vi "Select Channels and Update Properties.vi"(7 "guids":string[](array[string])=["4b95dee7-8d64-48ce-932c-f5fdd14e4d4c", "94e87467-031b-484c-a85e-bcbac581524d"], 8 "error in (no error)":errorcluster, 11 "Node Ptr":u64) -> (0 "error out":errorcluster)   [LabVIEW 2019, in "Protection and Counter Support System Explorer.lvlib"]
uses:
  Protection and Counter Support System Explorer.lvlib
  <vilib>/NI VeriStand/Custom Device Tools/Custom Device Utility Library/Custom Device Utility Library.lvlib
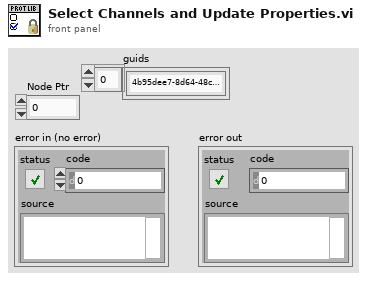
[diagram p1: front panel]
types:
  T1 = typedef "Protection and Counter Support System Explorer.lvlib/Protection Signal Settings.ctl" = cluster{"Input Channels":T2[], "Protection Type":T4}
  T2 = typedef "Protection and Counter Support System Explorer.lvlib/Protection Signal Linked Channel.ctl" = cluster{"Node Ref":T3}
  T3 = typedef "Custom Device API.lvlib/Custom Device Item Ref.ctl" = u64
  T4 = typedef "Protection and Counter Support Shared.lvlib/Protection Type.ctl" = enum16{"Arb ID + Bytes Checksum with Inversion", "Arb ID + Bytes CRC with Inversion", "Reversed Raw Signal Checksum with Inversion", "Concatenated Two's Compliment"}
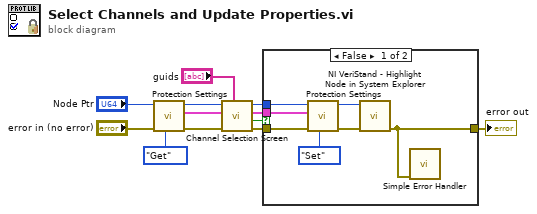
[diagram p0: block diagram]
diagram:
  n1 = call "Protection Settings.vi"("Action"=enum8{"Get", "Set"}."Get", "error in"="error in (no error)", "Parent Ref"="Node Ptr") -> ("error out"=w4:errorcluster, "Selected Channels"=w11:T1, "Parent Ref Out"=w3:T3)  [unwired: 6 in]
  n2 = call "Channel Selection Screen.vi"("guids"="guids", "error in"=w4, "Selected Channels"=w11, "Parent Ref"=w3) -> ("error out"=w6:errorcluster, "Cancelled?"=w8:bool, "Selected Channels"=w12:T1, "Parent Ref Out"=w7:T3)  [unwired: 4 in]
  n3 = case shown="False" w8 {
    tunnel: w6 -> [w16 w20]
    tunnel: w7 -> [w14 _]
    tunnel: w12 -> [w15 _]
    tunnel: [w17 w20] -> w10
    frame False {
      n4 = call "Protection Settings.vi"("Action"=enum8{"Get", "Set"}."Set", "error in"=w16, "Selected Channels"=w15, "Parent Ref"=w14) -> ("error out"=w18:errorcluster, "Parent Ref Out"=w19:T3)  [unwired: 5 in, 1 out]
      n5 = call <vilib>:"NI VeriStand - Highlight Node in System Explorer.vi"("error in (no error)"=w18, "Item Ref in"=w19) -> ("error out"=w17:errorcluster)  [unwired: 8 in, 1 out]
      n6 = call <vilib>:"Simple Error Handler.vi"("error in (no error)"=w17) -> ()  [unwired: 4 in, 5 out]
    }
    frame True {
    }
  }
  "error out" <- w10
